vi "Icon File Stem.vi"(8 "Error In":errorcluster, 10 "Indicator":bool, 11 "Value":variant) -> (0 "Error Out":errorcluster, 3 "String":string)   [LabVIEW 2018, in "Scripts.lvlib"]
uses:
  Scripts.lvlib
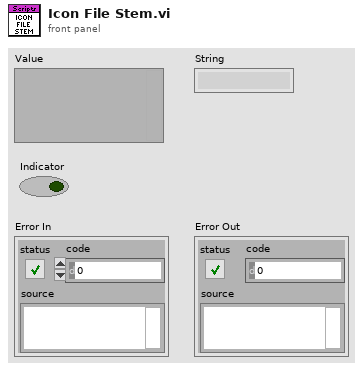
[diagram p1: front panel]
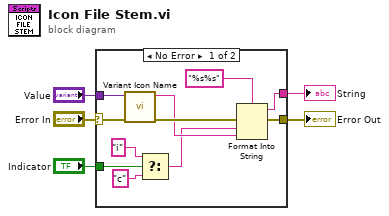
[diagram p0: block diagram]
diagram:
  n1 = case shown="No Error" "Error In" {
    selector: "Error In" -> [w6 w17]
    tunnel: [w16 _] -> w5
    tunnel: "Value" -> [w15 _]
    tunnel: [w12 w17] -> w3
    tunnel: "Indicator" -> [w7 _]
    frame No Error {
      n2 = call "Variant Icon Name.vi"("Error In"=w6, "Value"=w15) -> ("Error Out"=w14:errorcluster, "String"=w13:string)  [unwired: 8 in]
      n3 = Select(t="i", s=w7, f="c") -> (s? t:f=w10:string)
      n4 = Format Into String(format string="%s%s", error in=w14, w10, w13) -> (resulting string=w16:string, error out=w12:errorcluster)  [unwired: 1 in]
    }
    frame Error {
    }
  }
  "String" <- w5
  "Error Out" <- w3
